vi "poling.vi"() -> ()   [LabVIEW 2013]
uses:
  Rinocloud Library.lvlib
panel:
  in  "stop":bool
  out "active item name":string
  in  "active directory ID":string
  in  "new":bool
  in  "New folder name":string
  in  "Children":string(tree)
  in  "Ancestors":string(tree)
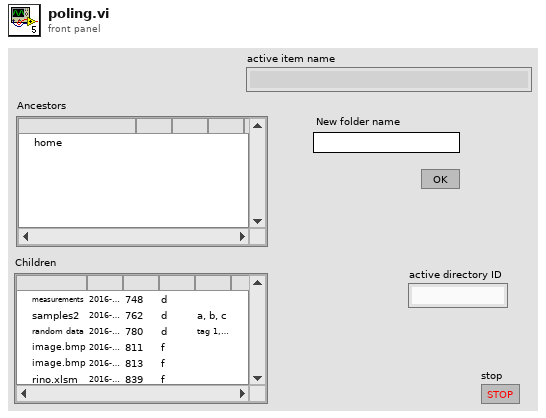
[diagram p1: front panel]
types:
  T1 = cluster{"name":string, "tags":string, "notes":string, "custom metadata array":cluster{"Attribute":string, "Value":string, "Data type":u16}[]}
  T2 = cluster{"active directory ID":string, "active file ID":string, "active object ID":string, "recent ID":string, "active item name":string}
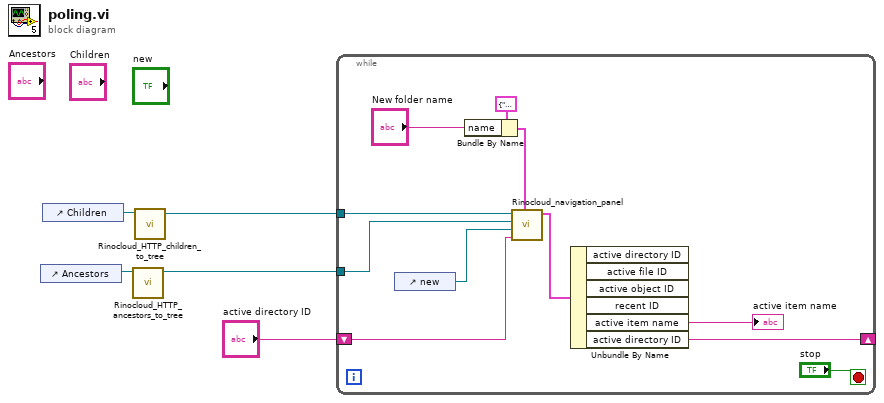
[diagram p0: block diagram]
diagram:
  n1 = control-ref of="Ancestors"() -> (w5:refnum<vi>)
  n2 = control-ref of="Children"() -> (w3:refnum<vi>)
  n3 = call "Rinocloud_HTTP_ancestors_to_tree.vi"("Tree Ref in"=w5) -> ("Tree Ref out"=w4:refnum<vi>)  [unwired: 3 in, 3 out]
  n4 = call "Rinocloud_HTTP_children_to_tree.vi"("Tree Ref in"=w3) -> ("Tree Ref out"=w2:refnum<vi>)  [unwired: 2 in, 2 out]
  n5 = while {
    tunnel: w4 -> [w9]
    tunnel: w2 -> [w8]
    shift-right: [w6] -> _
    shift-left: "active directory ID" -> [w7]
    stop <- "stop" stop-if-true
    n6 = control-ref of="new"() -> (w16:refnum<vi>)
    n7 = Bundle By Name(cluster=T1 {"name"="", "tags"="", "notes"="", "custom metadata array"=[]} ("metadata"), "name"="New folder name") -> (w11:T1)
    n8 = call "Rinocloud_navigation_panel.vi"("metadata"=w11, "active directory ID"=w7, "new folder ref"=w16, "ancestor tree ref"=w9, "children tree ref"=w8) -> ("active items"=w15:T2)  [unwired: 6 in]
    n9 = Unbundle By Name(w15) -> ("active item name"=→"active item name":string, "active directory ID"=w6:string)  [unwired: 4 out]
  }
